vi "Octave band frequencies.vi"(0 "octave band selector":i32, 1 "reference frequency range":u16(ring)=1 items=["Infrasonic", "Audio", "Ultrasonic"], 4 "bandwidth":T2(ring), 5 "standard":T1) -> (2 "reference frequency [Hz]":dbl format="%.2f", 3 "bandedge frequencies [Hz]":cluster{"f low":dbl, "f high":dbl} {"f high" format="%.2f"; "f low" format="%.2f"}, 6 "bandwidth designator":dbl format="%.2f", 7 "midband frequency [Hz]":dbl format="%.2f")   [LabVIEW 2017]
doc: "Returns the midband and bandedge frequencies associated with a particular fractional-octave band based on the specified bandwidth and standard (ANSI or IEC).\nThe octave band selector specifies the fractional-octave band. A value of 0 corresponds to the reference frequency of the audio-frequency range, 1 kHz. Each successive value corresponds to the next fractional-octave band. Positive values cover the range above 1 kHz, and negative values cover the range below 1 kHz."
uses:
  <vilib>/addons/_NISVFA/_Shared subVIs/Controls/svc_Octave Standard.ctl
  <vilib>/addons/Sound and Vibration/svt_Octave/SoundVib_Octave.lvlib
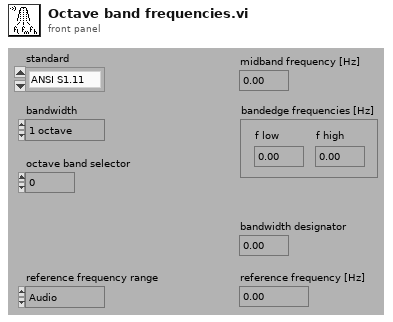
[diagram p1: front panel]
types:
  T1 = typedef "svc_Octave Standard.ctl" = enum16{"ANSI S1.11", "IEC 61260"}
  T2 = enum16{"1 octave", "1/3 octave", "1/6 octave", "1/12 octave", "1/24 octave"}
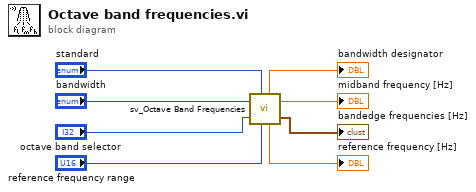
[diagram p0: block diagram]
diagram:
  n1 = call <vilib>:"sv_Octave Band Frequencies.vi"("octave band selector"="octave band selector", "reference frequency range"="reference frequency range", "bandwidth"="bandwidth", "standard"="standard") -> ("reference frequency [Hz]"=→"reference frequency [Hz]":dbl, "bandedge frequencies [Hz]"=→"bandedge frequencies [Hz]":cluster{"f low":dbl, "f high":dbl}, "bandwidth designator"=→"bandwidth designator":dbl, "midband frequency [Hz]"=→"midband frequency [Hz]":dbl)
